vi "Rotork_Valve-2.vi"(8 "Array In 2":u8[](array[numeric])=[0, 0, 0, 0, 0, 0, 0], 9 "Array In 1":u8[](array[numeric])=[0, 0], 11 "Valve SP":u8[](array[numeric])=[0, 0]) -> (0 "Array Out 2":u8[](array[numeric]), 1 "Array Out 1":u8[](array[numeric]))   [LabVIEW 2014]
uses:
  <vilib>/rvi/eio/common/nirviEmuTemplateMethod_errors.vi
  <vilib>/eio/EIOMethodNode/EIOMethodNode.xnode
panel:
  # "Input"
  # "Output"
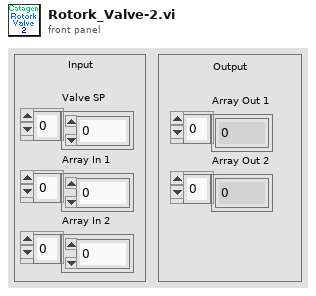
[diagram p1: front panel]
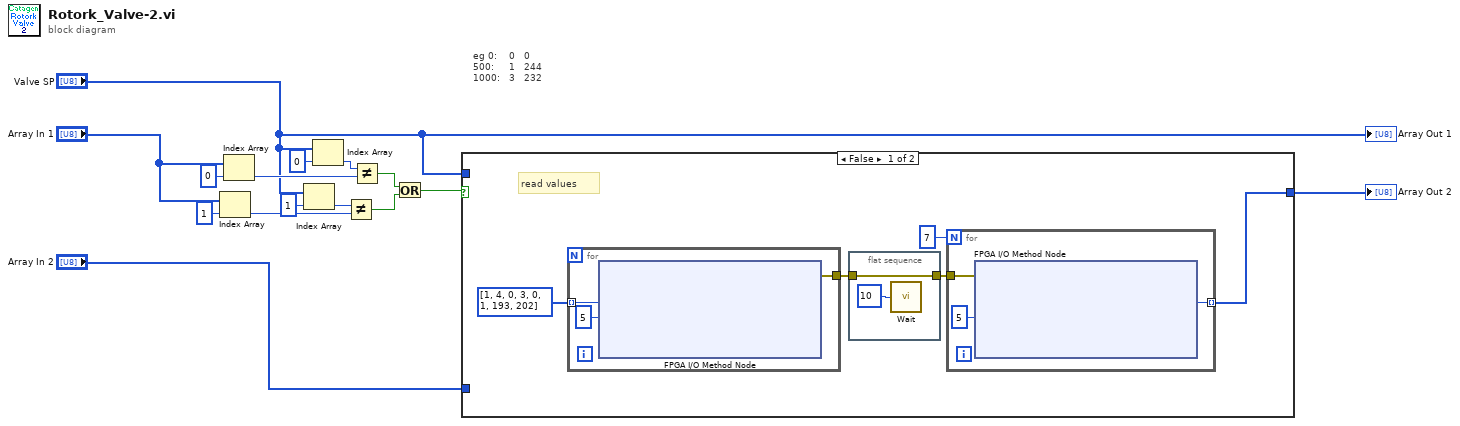
[diagram p0: block diagram]
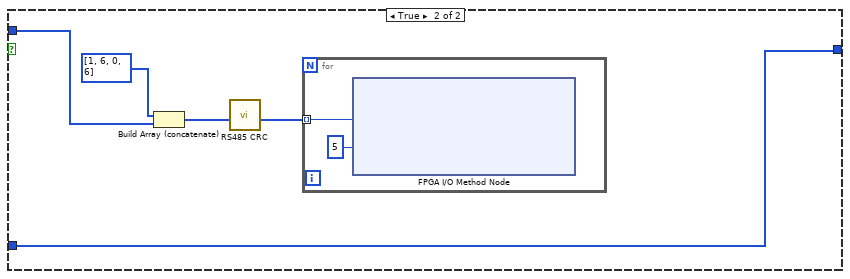
[diagram p2: hidden frame]
diagram:
  # "eg 0:    0   0\n500:     1   244\n1000:   3   232"
  n1 = Index Array(array="Array In 1", index=1) -> (element=w13:u8)
  n2 = Index Array(array="Array In 1", index=0) -> (element=w8:u8)
  n3 = Index Array(array="Valve SP", index=1) -> (element=w15:u8)
  n4 = Index Array(array="Valve SP", index=0) -> (element=w7:u8)
  n5 = Not Equal?(x=w15, y=w13) -> (x != y?=w12:bool)
  n6 = Not Equal?(x=w7, y=w8) -> (x != y?=w10:bool)
  n7 = Or(x=w10, y=w12) -> (x .or. y?=w9:bool)
  n8 = case shown="False" w9 {
    tunnel: [w16 w29] -> w2
    tunnel: "Array In 2" -> [_ w29]
    tunnel: "Valve SP" -> [_ w30]
    frame False {
      # "read values"
      n9 = for {
        tunnel: u8[] [1, 4, 0, 3, 0, 1, 193, 202] ("appended array") -> [w28] mode=indexing
        tunnel: [w26] -> w18
        n10 = xnode "FPGA I/O Method Node"("Data"=w28, "Timeout (ms)"=5) -> ("error out"=w26:errorcluster)  [unwired: 2 in, 2 out]
      }
      n11 = flat-sequence {
        tunnel: w18 -> [w24]
        tunnel: [w24] -> w19
        frame #0 {
          n12 = call "Wait"("Count(mSec)"=u32 10) -> ()  [unwired: 1 out]
        }
      }
      n13 = for {
        N: 7 -> [_]
        tunnel: w19 -> [w23]
        tunnel: [w22] -> w16 mode=indexing
        n14 = xnode "FPGA I/O Method Node"("error in"=w23, "Timeout (ms)"=5) -> ("Data"=w22:u8)  [unwired: 1 in, 3 out]
      }
    }
    frame True {
      n15 = Build Array (concatenate)(u8[] [1, 6, 0, 6] ("appended array"), w30) -> (w31:u8[])
      n16 = call "RS485 CRC.vi"("Data In"=w31) -> ("Data+CRC"=w33:u8[])  [unwired: 10 in]
      n17 = for {
        tunnel: w33 -> [w34] mode=indexing
        n18 = xnode "FPGA I/O Method Node"("Data"=w34, "Timeout (ms)"=5) -> ()  [unwired: 1 in, 2 out]
      }
    }
  }
  "Array Out 2" <- w2
  "Array Out 1" <- "Valve SP"
